vi "Write Actor Notifiers.vi"(10 "Base Actor Notifiers":T1, 11 "Template in":refnum<class "Template.lvclass">) -> (3 "Template out":refnum<class "Template.lvclass">)   [LabVIEW 2020, in "Template.lvlib" / "Template.lvclass"]
doc: "Sets the actor notifiers cluster"
uses:
  Template.lvclass
  typedefs/base actor notifiers.ctl
  Template.lvclass/Template.ctl
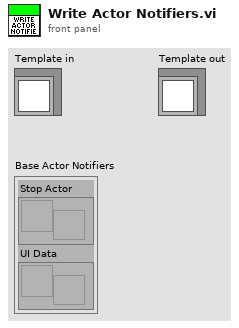
[diagram p1: front panel]
types:
  T1 = typedef "Template.lvlib/Template.lvclass/base actor notifiers.ctl" = cluster{"Stop Actor":refnum<notifier>, "UI Data":refnum<notifier>}
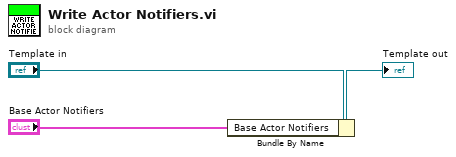
[diagram p0: block diagram]
diagram:
  n1 = Bundle By Name(cluster="Template in", "Base Actor Notifiers"="Base Actor Notifiers") -> (→"Template out":refnum<class "Template.lvclass">)
